vi "save_one_dat.vi"(8 "error in (no error)":errorcluster, 9 "modifier":string, 10 "type":string, 11 "dict of HIS IN":variant) -> (0 "error out":errorcluster, 3 "dict of HIS OUT":variant)   [LabVIEW 2020]
uses:
  cluster_template.ctl
  Classes/DATA/HIS/HIS.lvclass
  C:/dev/TRANCON/Classes/DATA/DATA.lvclass
  Classes/DATA/DATA.lvclass/DATA.ctl
  <vilib>/Utility/file.llb/Write Delimited Spreadsheet (DBL).vi
  Classes/DATA/DATA.lvclass
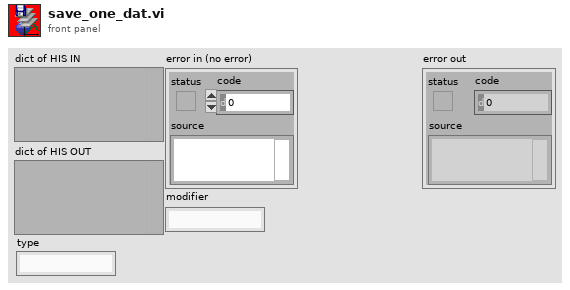
[diagram p1: front panel]
types:
  T1 = typedef "cluster_template.ctl" = cluster{"HIS.lvclass":refnum<class "HIS.lvclass">, "selector":refnum<vi>, "HIS graph":refnum<vi>, "DAT graph":refnum<vi>, "path":refnum<vi>, "path MAIN":refnum<vi>, "#":refnum<vi>, "unsel Graph":refnum<vi>, "DATgraph":refnum<vi>}
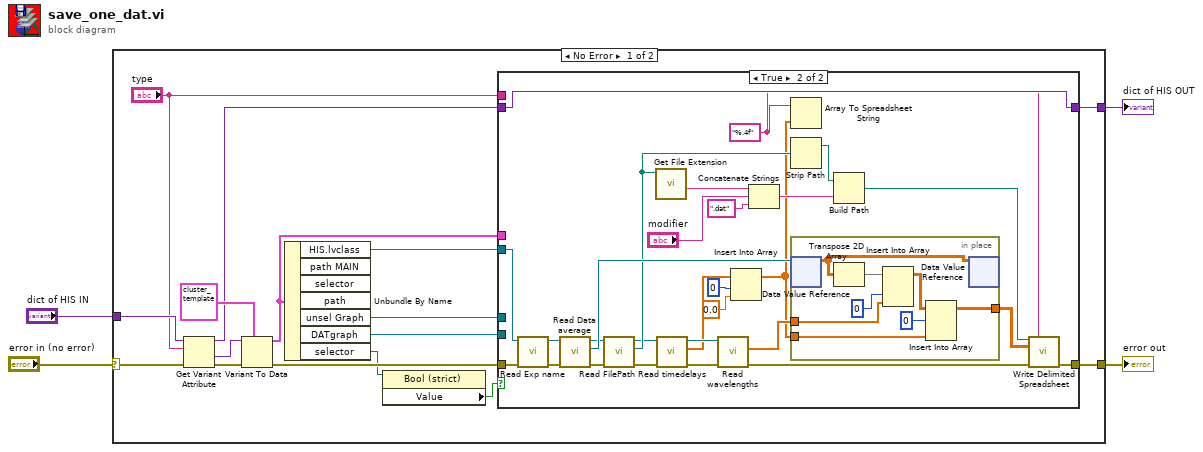
[diagram p0: block diagram]
diagram:
  n1 = case shown="No Error" "error in (no error)" {
    selector: "error in (no error)" -> [w19 w60]
    tunnel: "dict of HIS IN" -> [w20 w59]
    tunnel: [w14 w59] -> w3
    tunnel: [w5 w60] -> w2
    frame No Error {
      n2 = Get Variant Attribute(Variant=w20, name="type", error in=w19) -> (duplicate Variant=w13:variant, value=w18:variant, error out=w17:errorcluster)  [unwired: 1 in, 1 out]
      n3 = Variant To Data(error in=w17, type=T1 {"HIS.lvclass"=refnum, "selector"=refnum, "HIS graph"=refnum, "DAT graph"=refnum, "path"=refnum, "path MAIN"=refnum, "#"=refnum, "unsel Graph"=refnum, "DATgraph"=refnum} ("output cluster"), Variant=w18) -> (data=w15:T1, error out=w10:errorcluster)
      n4 = Unbundle By Name(w15) -> ("HIS.lvclass"=w9:refnum<class "HIS.lvclass">, "unsel Graph"=w11:refnum<vi>, "DATgraph"=w8:refnum<vi>, "selector"=w7:refnum<vi>)  [unwired: 3 out]
      n5 = property class="Bool (strict)"(reference=w7) -> ("Value"=w6:bool)  [unwired: 1 in, 2 out]
      n6 = case shown="True" w6 {
        tunnel: w15 -> [_ _]
        tunnel: [w22 w43] -> w14
        tunnel: w13 -> [w22 w43]
        tunnel: "type" -> [_ _]
        tunnel: w11 -> [_ _]
        tunnel: w10 -> [w21 w50]
        tunnel: w9 -> [_ w49]
        tunnel: w8 -> [_ _]
        tunnel: [w21 w24] -> w5
        frame False {
        }
        frame True {
          w26 = "%.4f" ("format string")
          n7 = call "Read Exp name.vi"("error in (no error)"=w50, "DATA in"=w49) -> ("error out"=w48:errorcluster, "DATA out"=w47:refnum<class "HIS.lvclass">)  [unwired: 7 in, 1 out]
          n8 = call "Read Data average.vi"("error in (no error)"=w48, "DATA in"=w47) -> ("error out"=w45:errorcluster, "Data average"=w46:refnum<data-value>, "DATA out"=w44:refnum<class "HIS.lvclass">)  [unwired: 7 in]
          n9 = call "Read FilePath.vi"("error in (no error)"=w45, "DATA in"=w44) -> ("error out"=w36:errorcluster, "FilePath"=w41:path, "DATA out"=w35:refnum<class "HIS.lvclass">)  [unwired: 7 in]
          n10 = call <vilib>:"Get File Extension.vi"("file"=w41) -> ("filename without extension"=w40:string)  [unwired: 6 in, 4 out]
          n11 = call "Read timedelays.vi"("error in (no error)"=w36, "DATA in"=w35) -> ("error out"=w34:errorcluster, "timedelays"=w32:dbl[], "DATA out"=w33:refnum<class "HIS.lvclass">)  [unwired: 7 in]
          n12 = call "Read wavelengths.vi"("error in (no error)"=w34, "DATA in"=w33) -> ("error out"=w25:errorcluster, "wavelengths"=w29:dbl[])  [unwired: 7 in, 1 out]
          n13 = Insert Into Array(array=w32, index=0, new element=0.0 ("new element/subarray")) -> (w28:dbl[])
          n14 = Concatenate Strings(w40, "modifier", ".dat" ("string")) -> (w37:string)
          n15 = Array To Spreadsheet String(array=w28, 3:w26) -> ()  [unwired: 1 in, 1 out]
          n16 = Strip Path(path=w41) -> (stripped path=w42:path)  [unwired: 1 out]
          n17 = in-place {
            in-place-border: w29 -> [w56]
            in-place-border: w28 -> [w53]
            in-place-border: [w52] -> w27
            n18 = in-place-dvr #1(w46) -> (w58:dbl[][])  [unwired: 1 out]
            n19 = Transpose 2D Array(2D array=w58) -> (transposed array=w51:dbl[][])
            n20 = Insert Into Array(array=w51, index (col)=0 ("disabled index (col)"), new element=w56) -> (w55:dbl[][])  [unwired: 1 in]
            n21 = Insert Into Array(array=w55, index (row)=0, new element=w53) -> (w52:dbl[][])  [unwired: 1 in]
            n22 = in-place-dvr #1(w58) -> ()  [unwired: 2 out]
          }
          n23 = Build Path(base path=w42, name or relative path=w37) -> (appended path=w23:path)
          n24 = call-poly <vilib>:"Write Delimited Spreadsheet.vi"("file path (dialog if empty)"=w23, "format (%.3f)"=w26, "2D data"=w27, "error in (no error)"=w25) -> ("error out"=w24:errorcluster)  [unwired: 10 in, 1 out]
        }
      }
    }
    frame Error {
    }
  }
  "dict of HIS OUT" <- w3
  "error out" <- w2
